vi "Drive Controller.vi"(8 "error in":errorcluster) -> ()   [LabVIEW 2019]
doc: "This VI executes continuously carrying out the current operation and responding to updates or new operation requests. It will often contain the timing or control code that is difficult to place directly in TeleOp. This VI generally opens all sensors and motors and isolates the rest of the robot code from knowing implementation details of how the operations are carried out."
uses:
  <vilib>/Rock Robotics/WPI/Framework/Completion Status.ctl
  Drive Setpoints.ctl
  Drive Operations.ctl
  <vilib>/Rock Robotics/WPI/SafetyOutput/WPI_SafetyOutputConfigMenu.ctl
  <vilib>/Rock Robotics/WPI/RobotDrive/WPI_RobotDriveDevRef.ctl
  <vilib>/Rock Robotics/WPI/MotorControl/WPI_MotorControlDeviceRef.ctl
  <vilib>/Rock Robotics/WPI/MotorControl/WPI_MotorControlType.ctl
  <vilib>/Rock Robotics/SystemInterfaces/DIO/FPGA_DIOPWMChannel.ctl
  <vilib>/Rock Robotics/WPI/PWM/WPI_PWMDeadband.ctl
  <vilib>/Rock Robotics/SystemInterfaces/DIO/FPGA_DIOChannel.ctl
  InitialHeading.vi
  <vilib>/Rock Robotics/WPI/RobotDrive/WPI_RobotDriveMecanumDrive_Cartesian.vi
  <vilib>/Rock Robotics/Network Tables/NT Read Number.vi
  DistanceToTarget.vi
panel:
  out "YRPHfH 2":T1
  out "left motors":dbl
  out "right motors":dbl
  out "YRPHfH":T1
  in  "Interactive Values":T2
  in  "Buttons":cluster{"Execute Cmd":bool, "Abort Cmd":bool}
  out "Command Timing":cluster{"Start Time (ms)":u32, "Iterations":i32}
  out "Status":T4
  out "Current\nCmd":string
  # "Tip: The graph shows the motor setpoints. It may also be helpful to observe inputs and sensor values.\nYou may also want to display tuning or debugging controls."
  # "Interactive Command: You may fill in the settings for a command\nand schedule it with the Execute button. You can observe and abort\nany command while fine tuning the code for the controller."
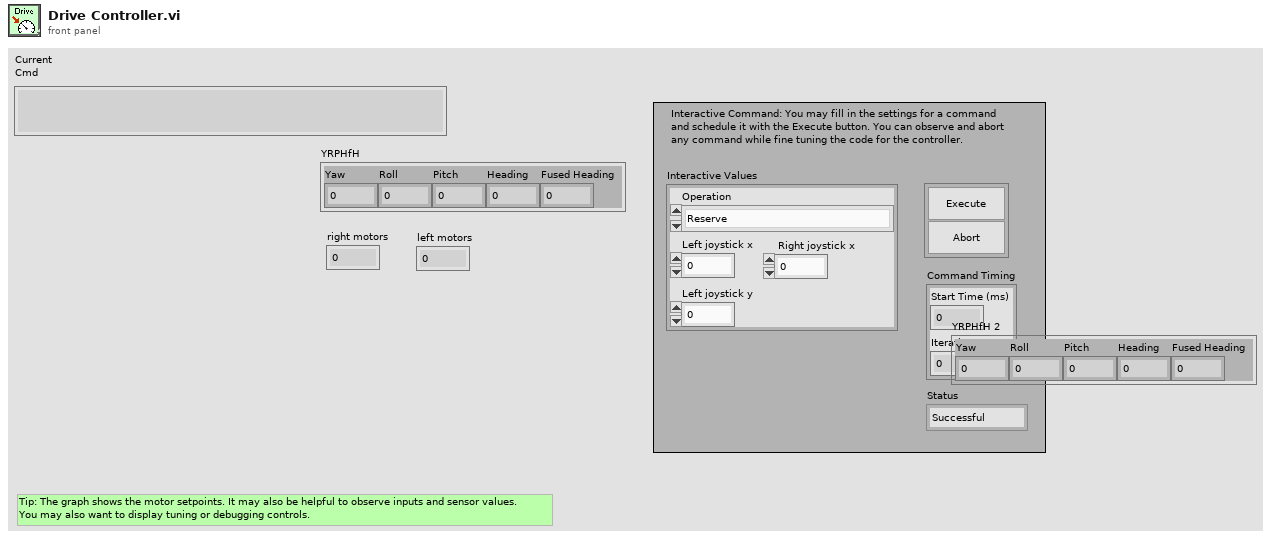
[diagram p1: front panel]
types:
  T1 = cluster{"Yaw":dbl, "Roll":dbl, "Pitch":dbl, "Heading":dbl, "Fused Heading":dbl}
  T2 = typedef "Drive Setpoints.ctl" = cluster{"Operation":T3, "Left joystick x":dbl, " Right joystick x":dbl, "Left joystick y":dbl}
  T3 = typedef "Drive Operations.ctl" = enum16{"Reserve", "Sniper Drive", "Set Initial Heading", "Read Current", "Immediate", "Drive for Time", "Drive for Distance"}
  T4 = typedef "Completion Status.ctl" = enum16{"Successful", "Aborted", "Incomplete"}
  T5 = typedef "WPI_RobotDriveDevRef.ctl" = cluster{"DevStatus":errorcluster, "Motors[]":T6[], "Square Inputs":bool, "Max Output":dbl}
  T6 = typedef "WPI_MotorControlDeviceRef.ctl" = cluster{"DeviceStatus":errorcluster, "Type":T7, "PWM":cluster{"PWM Channel":T8, "DeadBand":T9}, "CAN":cluster{"Device Number":u8, "SetOutput VI Ref":variant, "GetOutput VI Ref":variant, "Enable VI Ref":variant, "Disable VI Ref":variant, "Data":variant}, "Invert":bool, "DIO PWM":cluster{"PWM \"Enable\" Channel":T8, "DIOChannel":T10, "PWM Rate":dbl}}
  T7 = typedef "WPI_MotorControlType.ctl" = enum16{"PWM", "CAN", "DIO PWM"}
  T8 = typedef "FPGA_DIOPWMChannel.ctl" = enum8{"PWM 0", "PWM 1", "PWM 2", "PWM 3", "PWM 4", "PWM 5", "PWM 6", "PWM 7", "PWM 8", "PWM 9", "PWM MXP 0", "PWM MXP 1", "PWM MXP 2", "PWM MXP 3", "PWM MXP 4", "PWM MXP 5", "PWM MXP 6", "PWM MXP 7", "PWM MXP 8", "PWM MXP 9", "Invalid"}
  T9 = typedef "WPI_PWMDeadband.ctl" = cluster{"Name":string, "maxPositivePwm":i32, "minPositivePwm":i32, "centerPwm":i32, "maxNegativePwm":i32, "minNegativePwm":i32, "angularRange":u16}
  T10 = typedef "FPGA_DIOChannel.ctl" = enum8{"DIO 0", "DIO 1", "DIO 2", "DIO 3", "DIO 4", "DIO 5", "DIO 6", "DIO 7", "DIO 8", "DIO 9", "DIO MXP 0", "DIO MXP 1", "DIO MXP 2", "DIO MXP 3", "DIO MXP 4", "DIO MXP 5", "DIO MXP 6", "DIO MXP 7", "DIO MXP 8", "DIO MXP 9", "DIO MXP 10", "DIO MXP 11", "DIO MXP 12", "DIO MXP 13", "DIO MXP 14", "DIO MXP 15", "SPI Port CS1", "SPI Port CS2", "SPI Port CS3", "SPI Port MISO", "SPI Port MOSI", "Invalid"}
  T11 = typedef "WPI_SafetyOutputConfigMenu.ctl" = enum16{"Enable", "Disable"}
  T12 = typedef "Command Status Info.ctl" = cluster{"Name":string, "Status":T4, "notifier out":T13}
  T13 = typedef "Completion Notifier.ctl" = refnum<notifier>
  T14 = cluster{"SubSystem Data":T2, cluster{"Start Time (ms)":u32, "Iterations":i32}, cluster{"Command Info":T12, "Description":string, "Default Command":T2, "queue out":refnum<queue>, "Subsystem Name":string}}
  T15 = cluster{"SubSystem Data":T2, cluster{"Start Time (ms)":u32, "Iterations":i32}, "Default Command Arguments":cluster{"Command Info":T12, "Description":string, "Default Command":T2, "queue out":refnum<queue>, "Subsystem Name":string}}
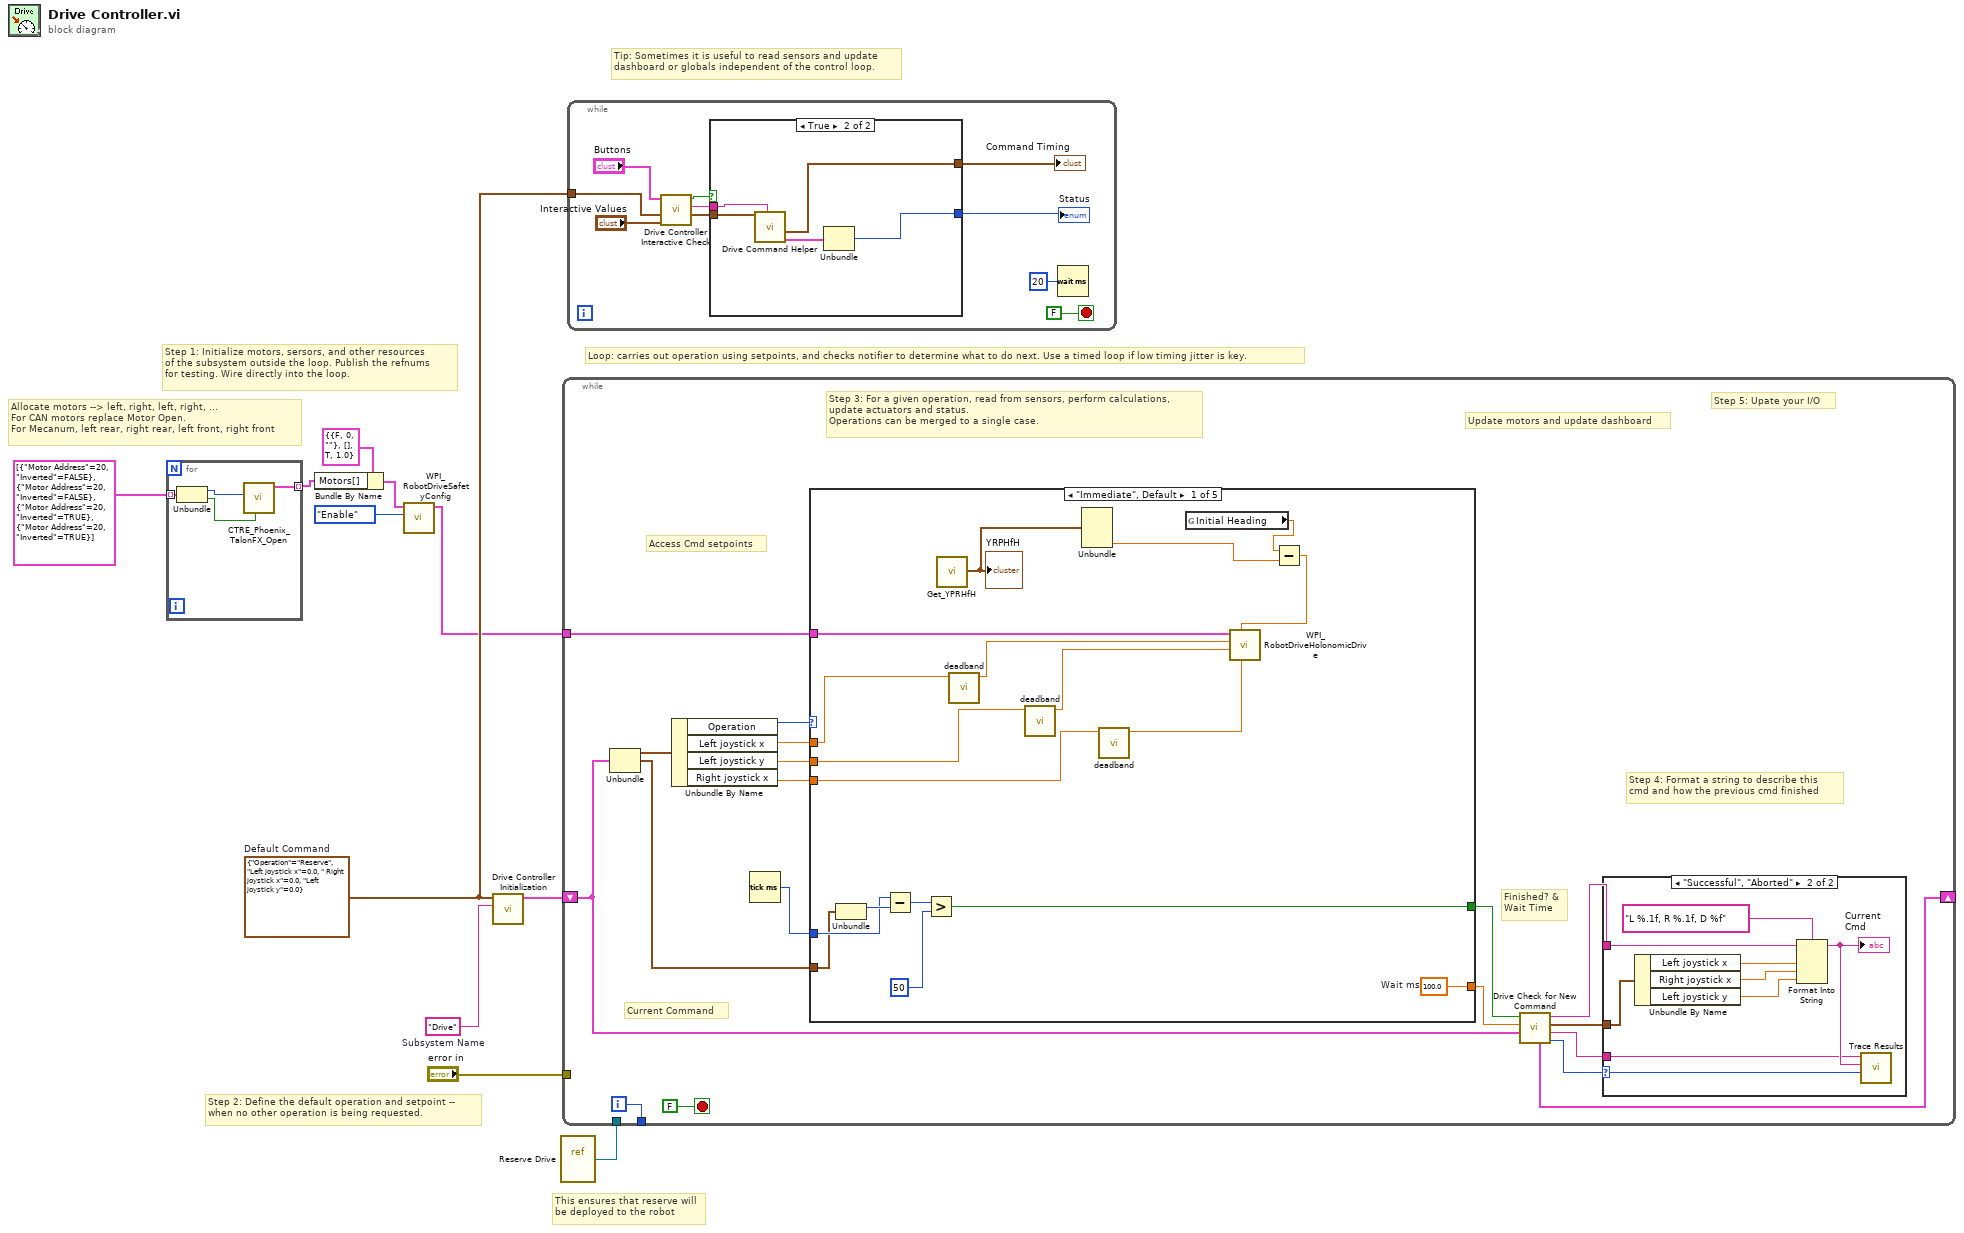
[diagram p0: block diagram]
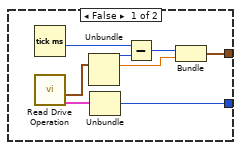
[diagram p2: hidden frame]
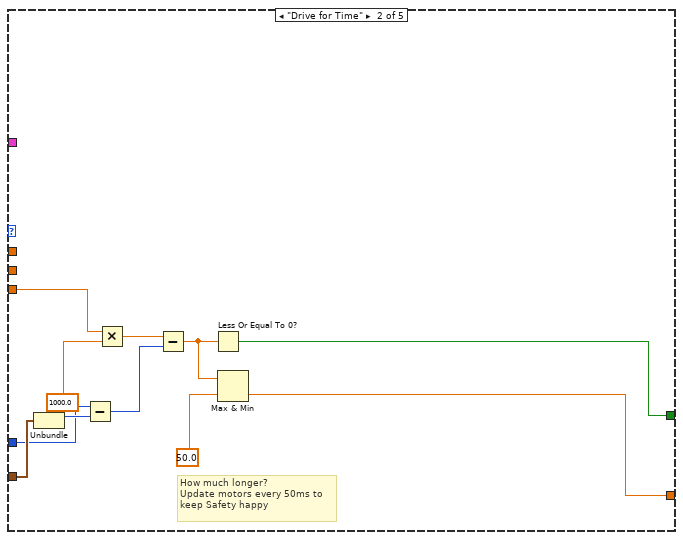
[diagram p4: hidden frame]
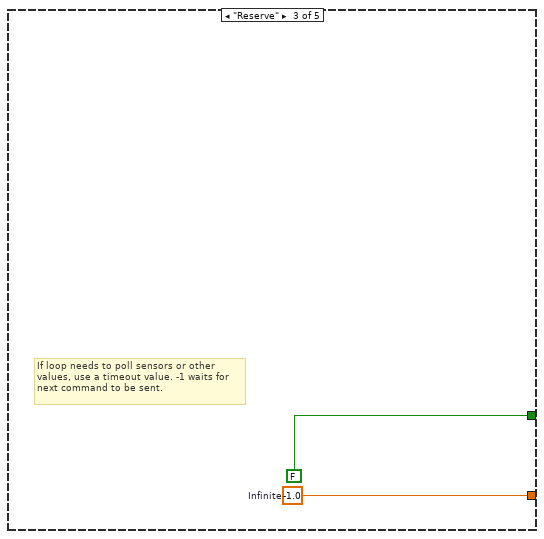
[diagram p5: hidden frame]
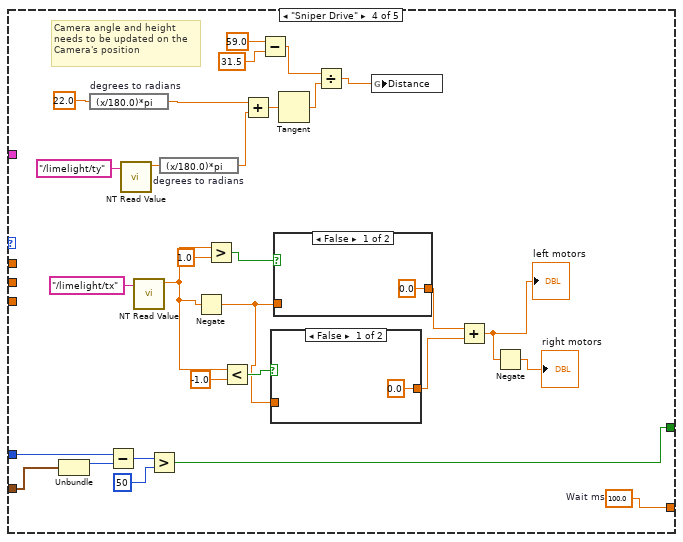
[diagram p6: hidden frame]
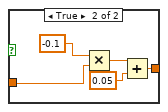
[diagram p7: hidden frame]
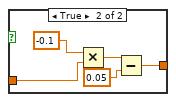
[diagram p8: hidden frame]
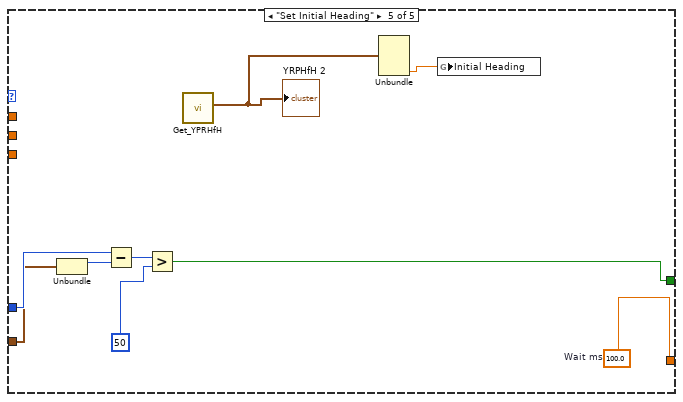
[diagram p9: hidden frame]
diagram:
  w7 = T2 {"Operation"=enum."Reserve", "Left joystick x"=0.0, " Right joystick x"=0.0, "Left joystick y"=0.0}  # Default Command
  w11 = "Drive"  # Subsystem Name
  # "Allocate motors --> left, right, left, right, ... \nFor CAN motors replace Motor Open.\nFor Mecanum, left rear, right rear, left front, right front"
  # "This ensures that reserve will\nbe deployed to the robot"
  # "Tip: Sometimes it is useful to read sensors and update\ndashboard or globals independent of the control loop."
  # "Step 2: Define the default operation and setpoint --\nwhen no other operation is being requested."
  # "Step 1: Initialize motors, sersors, and other resources\nof the subsystem outside the loop. Publish the refnums\nfor testing. Wire directly into the loop."
  # "Loop: carries out operation using setpoints, and checks notifier to determine what to do next. Use a timed loop if low timing jitter is key."
  n1 = for {
    tunnel: cluster{"Motor Address":i32, "Inverted":bool}[] [{"Motor Address"=20, "Inverted"=FALSE}, {"Motor Address"=20, "Inverted"=FALSE}, {"Motor Address"=20, "Inverted"=TRUE}, {"Motor Address"=20, "Inverted"=TRUE}] ("Array") -> [w15] mode=indexing
    tunnel: [w14] -> w3 mode=indexing
    n2 = Unbundle(w15) -> ("Motor Address"=w13:i32, "Inverted"=w12:bool)
    n3 = call <vilib>:"CTRE_Phoenix_TalonFX_Open.vi"("Invert"=w12, "Device Number"=w13) -> ("CAN Talon SRX Ref"=w14:T6)  [unwired: 8 in, 1 out]
  }
  n4 = Bundle By Name(cluster=T5 {"DevStatus"={"status"=FALSE, "code"=0, "source"=""}, "Motors[]"=[], "Square Inputs"=TRUE, "Max Output"=1.0} ("RobotDriveDevRef"), "Motors[]"=w3) -> (w6:T5)
  n5 = call <vilib>:"WPI_RobotDriveSafetyConfig.vi"("mode"=WPI_SafetyOutputConfigMenu."Enable", "RobotDriveDevRef"=w6) -> ("RobotDriveDevRef"=w1:T5)  [unwired: 2 in, 7 out]
  n6 = call "Drive Controller Initialization.vi"("Subsystem Name"=w11, "Default Command"=w7) -> ("Current Command"=w9:T14)  [unwired: 9 in]
  n7 = vi-ref "Reserve Drive.vi"() -> (w8:refnum<vi>)
  n8 = while {
    shift-right: [w24] -> _
    shift-left: w9 -> [w17]
    tunnel: [w32] -> _
    tunnel: "error in" -> [_]
    tunnel: w8 -> [_]
    tunnel: w1 -> [w16]
    i -> [w32]
    stop <- FALSE stop-if-true
    # "Step 5: Upate your I/O"
    # "Step 4: Format a string to describe this\ncmd and how the previous cmd finished"
    # "Current Command"
    # "Update motors and update dashboard"
    # "Access Cmd setpoints"
    # "Finished? &\nWait Time"
    # "Step 3: For a given operation, read from sensors, perform calculations,\nupdate actuators and status.\nOperations can be merged to a single case."
    n9 = Unbundle(w17) -> ("SubSystem Data"=w31:T2, w18:cluster{"Start Time (ms)":u32, "Iterations":i32})  [unwired: 1 out]
    n10 = Unbundle By Name(w31) -> ("Operation"=w30:T3, "Left joystick x"=w29:dbl, "Left joystick y"=w28:dbl, "Right joystick x"=w27:dbl)
    n11 = Tick Count (ms)() -> (millisecond timer value=w26:u32)
    n12 = case shown="\"Immediate\", Default" w30 {
      tunnel: [w60 w61 w73 w74 w118] -> w23
      tunnel: [w55 w66 FALSE ("ignore previous (F)") w75 w117] -> w22
      tunnel: w18 -> [w54 w68 _ w77 w119]
      tunnel: w29 -> [w46 _ _ _ _]
      tunnel: w28 -> [w45 _ _ _ _]
      tunnel: w27 -> [w44 w65 _ _ _]
      tunnel: w26 -> [w56 w64 _ w76 w120]
      tunnel: w16 -> [w47 _ _ _ _]
      frame "Immediate", Default {
        w60 = 100.0  # Wait ms
        n13 = Unbundle(w54) -> ("Start Time (ms)"=w57:u32)  [unwired: 1 out]
        n14 = Subtract(x=w56, y=w57) -> (x-y=w58:u32)
        n15 = Greater?(x=w58, y=u8 50 ("Left Motor")) -> (0:w55:bool)
        n16 = call <vilib>:"Get_YPRHfH.vi"() -> ("YRPHfH"=w50:T1)  [unwired: 11 in]
        "YRPHfH" <- w50
        n17 = call "deadband.vi"("Joystick Value"=w46) -> ("Val"=w51:dbl)  [unwired: 10 in]
        n18 = call "deadband.vi"("Joystick Value"=w45) -> ("Val"=w52:dbl)  [unwired: 10 in]
        n19 = Unbundle(w50) -> ("Fused Heading"=w49:dbl)  [unwired: 4 out]
        n20 = call "deadband.vi"("Joystick Value"=w44) -> ("Val"=w53:dbl)  [unwired: 10 in]
        n21 = global read "InitialHeading.vi" "Initial Heading"() -> (w43:dbl)
        n22 = Subtract(x=w43, y=w49) -> (x-y=w48:dbl)
        n23 = call-poly <vilib>:"WPI_RobotDriveHolonomicDrive.vi"("Rotation"=w53, "Gyro Angle"=w48, "Y"=w52, "X"=w51, "RobotDriveDevRef"=w47) -> ()  [unwired: 4 in, 3 out]
      }
      frame "Drive for Time" {
        # "How much longer?\nUpdate motors every 50ms to\nkeep Safety happy"
        n24 = Unbundle(w68) -> ("Start Time (ms)"=w67:u32)  [unwired: 1 out]
        n25 = Subtract(x=w64, y=w67) -> (x-y=w71:u32)
        n26 = Multiply(x=w65, y=1000.0) -> (x*y=w70:dbl)
        n27 = Subtract(x=w70, y=w71) -> (x-y=w63:dbl)
        n28 = Less Or Equal To 0?(x=w63) -> (x <= 0?=w66:bool)
        n29 = Max & Min(x=w63, y=50.0) -> (min(x,y)=w61:dbl)  [unwired: 1 out]
      }
      frame "Reserve" {
        w73 = -1.0  # Infinite
        # "If loop needs to poll sensors or other\nvalues, use a timeout value. -1 waits for\nnext command to be sent."
      }
      frame "Sniper Drive" {
        w74 = 100.0  # Wait ms
        # "Camera angle and height\nneeds to be updated on the\nCamera's position"
        n30 = Unbundle(w77) -> ("Start Time (ms)"=w78:u32)  [unwired: 1 out]
        n31 = expression code="(x/180.0)*pi" "degrees to radians"(22.0 ("x")) -> (w95:dbl)
        n32 = Subtract(x=w76, y=w78) -> (x-y=w79:u32)
        n33 = call-poly <vilib>:"NT Read Value.vi"("Name"="/limelight/ty") -> ("Numeric"=w98:dbl)  [unwired: 9 in, 1 out]
        n34 = call-poly <vilib>:"NT Read Value.vi"("Name"="/limelight/tx") -> ("Numeric"=w87:dbl)  [unwired: 9 in, 1 out]
        n35 = Greater?(x=w79, y=u8 50 ("Left Motor")) -> (0:w75:bool)
        n36 = expression code="(x/180.0)*pi" "degrees to radians"(w98) -> (w97:dbl)
        n37 = Negate(x=w87) -> (-x=w86:dbl)
        n38 = Greater?(x=w87, y=1.0) -> (0:w89:bool)
        n39 = Less?(x=w87, y=-1.0) -> (x < y?=w88:bool)
        n40 = Add(x=w95, y=w97) -> (x+y=w94:dbl)
        n41 = Subtract(x=59.0, y=31.5) -> (x-y=w99:dbl)
        n42 = case shown="False" w88 {
          tunnel: w86 -> [_ w105]
          tunnel: [0.0 w104] -> w84
          frame False {
          }
          frame True {
            n43 = Multiply(x=-0.1, y=w105) -> (x*y=w107:dbl)
            n44 = Add(x=w107, y=0.05) -> (x+y=w104:dbl)
          }
        }
        n45 = case shown="False" w89 {
          tunnel: w86 -> [_ w113]
          tunnel: [0.0 w110] -> w85
          frame False {
          }
          frame True {
            n46 = Multiply(x=-0.1, y=w113) -> (x*y=w112:dbl)
            n47 = Subtract(x=w112, y=0.05) -> (x-y=w110:dbl)
          }
        }
        n48 = Tangent(1:w94) -> (0:w93:dbl)
        n49 = Divide(x=w99, y=w93) -> (x/y=w81:dbl)
        n50 = global write "DistanceToTarget.vi" "Distance"(w81) -> ()
        n51 = Add(x=w85, y=w84) -> (x+y=w83:dbl)
        "left motors" <- w83
        n52 = Negate(x=w83) -> (-x=→"right motors":dbl)
      }
      frame "Set Initial Heading" {
        w118 = 100.0  # Wait ms
        n53 = Unbundle(w119) -> ("Start Time (ms)"=w121:u32)  [unwired: 1 out]
        n54 = Subtract(x=w120, y=w121) -> (x-y=w122:u32)
        n55 = Greater?(x=w122, y=u8 50 ("Left Motor")) -> (0:w117:bool)
        n56 = call <vilib>:"Get_YPRHfH.vi"() -> ("YRPHfH"=w116:T1)  [unwired: 11 in]
        "YRPHfH 2" <- w116
        n57 = Unbundle(w116) -> ("Fused Heading"=w115:dbl)  [unwired: 4 out]
        n58 = global write "InitialHeading.vi" "Initial Heading"(w115) -> ()
      }
    }
    n59 = call "Drive Check for New Command.vi"("input cluster"=w17, "Wait time (ms)"=w23, "Finished?"=w22) -> ("Completion"=w25:T4, "Subsystem Name"=w19:string, "Current Command"=w20:T2, "Initial Trace String"=w21:string, "Next Command"=w24:T15)  [unwired: 4 in]
    n60 = case shown="\"Successful\", \"Aborted\"" w25 {
      selector: w25 -> [_ w42]
      tunnel: w21 -> [_ w37]
      tunnel: w20 -> [_ w38]
      tunnel: w19 -> [_ w34]
      frame "Incomplete", Default {
        # "Continuing current command"
      }
      frame "Successful", "Aborted" {
        # "Report and setup for next command"
        n61 = Unbundle By Name(w38) -> ("Left joystick x"=w40:dbl, "Right joystick x"=w41:dbl, "Left joystick y"=w35:dbl)
        n62 = Format Into String(format string="L %.1f, R %.1f, D %f", initial string=w37, w40, w41, w35) -> (resulting string=w36:string)  [unwired: 1 in, 1 out]
        "Current\nCmd" <- w36
        n63 = call <vilib>:"Trace Results.vi"("Status of previous command"=w42, "Description"=w36, "Subsystem"=w34) -> ()  [unwired: 9 in]
      }
    }
  }
  n64 = while {
    tunnel: w7 -> [w125]
    stop <- FALSE stop-if-true
    n65 = call "Drive Controller Interactive Check.vi"("Interactive Command In"="Interactive Values", "Default Command"=w125, "Buttons"="Buttons") -> ("Interactive Command Out"=w127:T2, "Trace String"=w128:string, "Schedule"=w129:bool)  [unwired: 6 in]
    n66 = case shown="True" w129 {
      tunnel: [w138 w146] -> w130
      tunnel: [w137 w142] -> w131
      tunnel: w128 -> [_ w144]
      tunnel: w127 -> [_ w143]
      frame False {
        n67 = Tick Count (ms)() -> (millisecond timer value=w141:u32)
        n68 = call "Read Drive Operation.vi"() -> ("Command Info"=w135:T12, "SubSystem Data"=w134:T2)  [unwired: 9 in, 1 out]
        n69 = Unbundle(w134) -> ("Operation"=w139:T3, "Left joystick x"=w136:dbl)  [unwired: 2 out]
        n70 = Unbundle(w135) -> ("Status"=w138:T4)  [unwired: 2 out]
        n71 = Subtract(x=w141, y=w139) -> (x-y=w140:u32)
        n72 = Bundle(w140, "Left joystick x"=w136) -> (w137:cluster{u32, "Left joystick x":dbl})  [unwired: 1 in]
      }
      frame True {
        n73 = call "Drive Command Helper.vi"("Description"=w144, "SubSystem Data"=w143) -> ("Command Info Out"=w145:T12, "Command Timing"=w142:cluster{"Start Time (ms)":u32, "Iterations":i32})  [unwired: 7 in, 1 out]
        n74 = Unbundle(w145) -> ("Status"=w146:T4)  [unwired: 2 out]
      }
    }
    "Status" <- w130
    "Command Timing" <- w131
    n75 = Wait (ms)(milliseconds to wait=u32 20) -> ()  [unwired: 1 out]
  }
